vi "Init_PathPoints_Queue.vi"(8 "error in (no error)":errorcluster) -> (0 "error out":errorcluster, 2 "Q_Ref_Out":T1)   [LabVIEW 2017]
doc: "Initialise notifiers and queues"
uses:
  Ctl/Q_Ref_Cluster.ctl
  Ctl/Current_Position.ctl
  Ctl/Mapping_Sensor_Data.ctl
  ROS/LaserScan.ctl
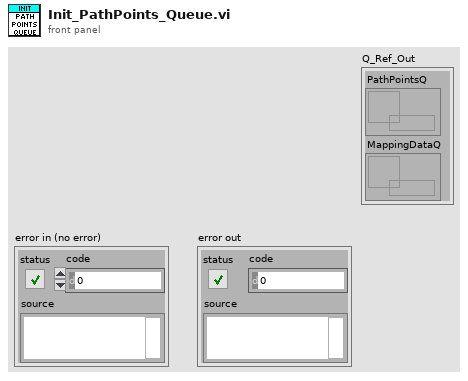
[diagram p1: front panel]
types:
  T1 = typedef "Q_Ref_Cluster.ctl" = cluster{"PathPointsQ":refnum<queue>, "MappingDataQ":refnum<queue>}
  T2 = typedef "Current_Position.ctl" = cluster{"X":dbl, "Y":dbl, "Theta":dbl}
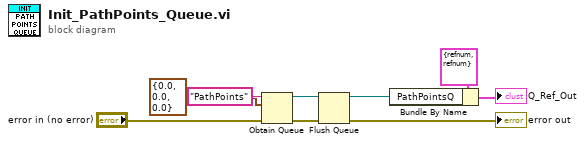
[diagram p0: block diagram]
diagram:
  n1 = Obtain Queue(name (unnamed)="PathPoints", element data type=T2 {"X"=0.0, "Y"=0.0, "Theta"=0.0} ("Current_Position_in"), error in (no error)="error in (no error)") -> (queue out=w3:refnum<queue>, error out=w7:errorcluster)  [unwired: 2 in, 1 out]
  n2 = Flush Queue(queue=w3, error in (no error)=w7) -> (queue out=w2:refnum<queue>, error out=→"error out":errorcluster)  [unwired: 1 out]
  n3 = Bundle By Name(cluster=T1 {"PathPointsQ"=refnum, "MappingDataQ"=refnum} ("Q_Ref_Cluster"), "PathPointsQ"=w2) -> (→"Q_Ref_Out":T1)
